vi "example_microFPGA_TTL.vi"() -> ()   [LabVIEW 2021]
panel:
  out "TTL_mode_READ":u16(ring)=1 items=["LO", "HIGH"]
  in  "TTL_channel":u16(ring)=3 items=["channel No 0", "channel No 1", "channel No 2", "channel No 3"]
  in  "write or read":u16(ring)=1 items=["read", "write"]
  out "value confirm":bool
  out "Version":u16=3
  in  "TTL_channel_WRITE":u16(ring)=1 items=["LO", "HIGH"]
  in  "close Application":bool=TRUE
  in  "send parameters":bool
  # "TTL control"
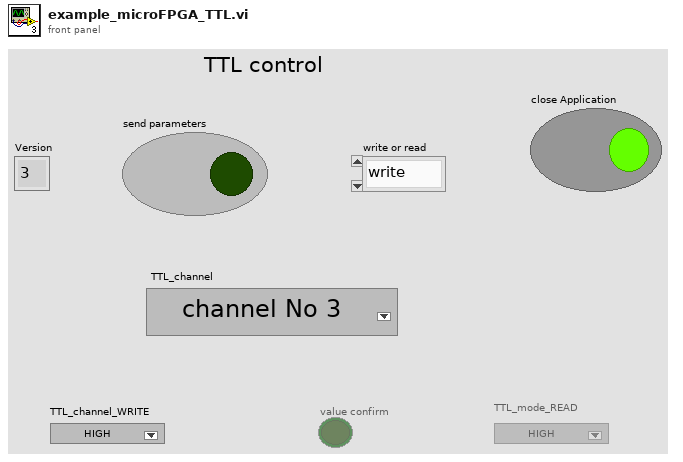
[diagram p1: front panel]
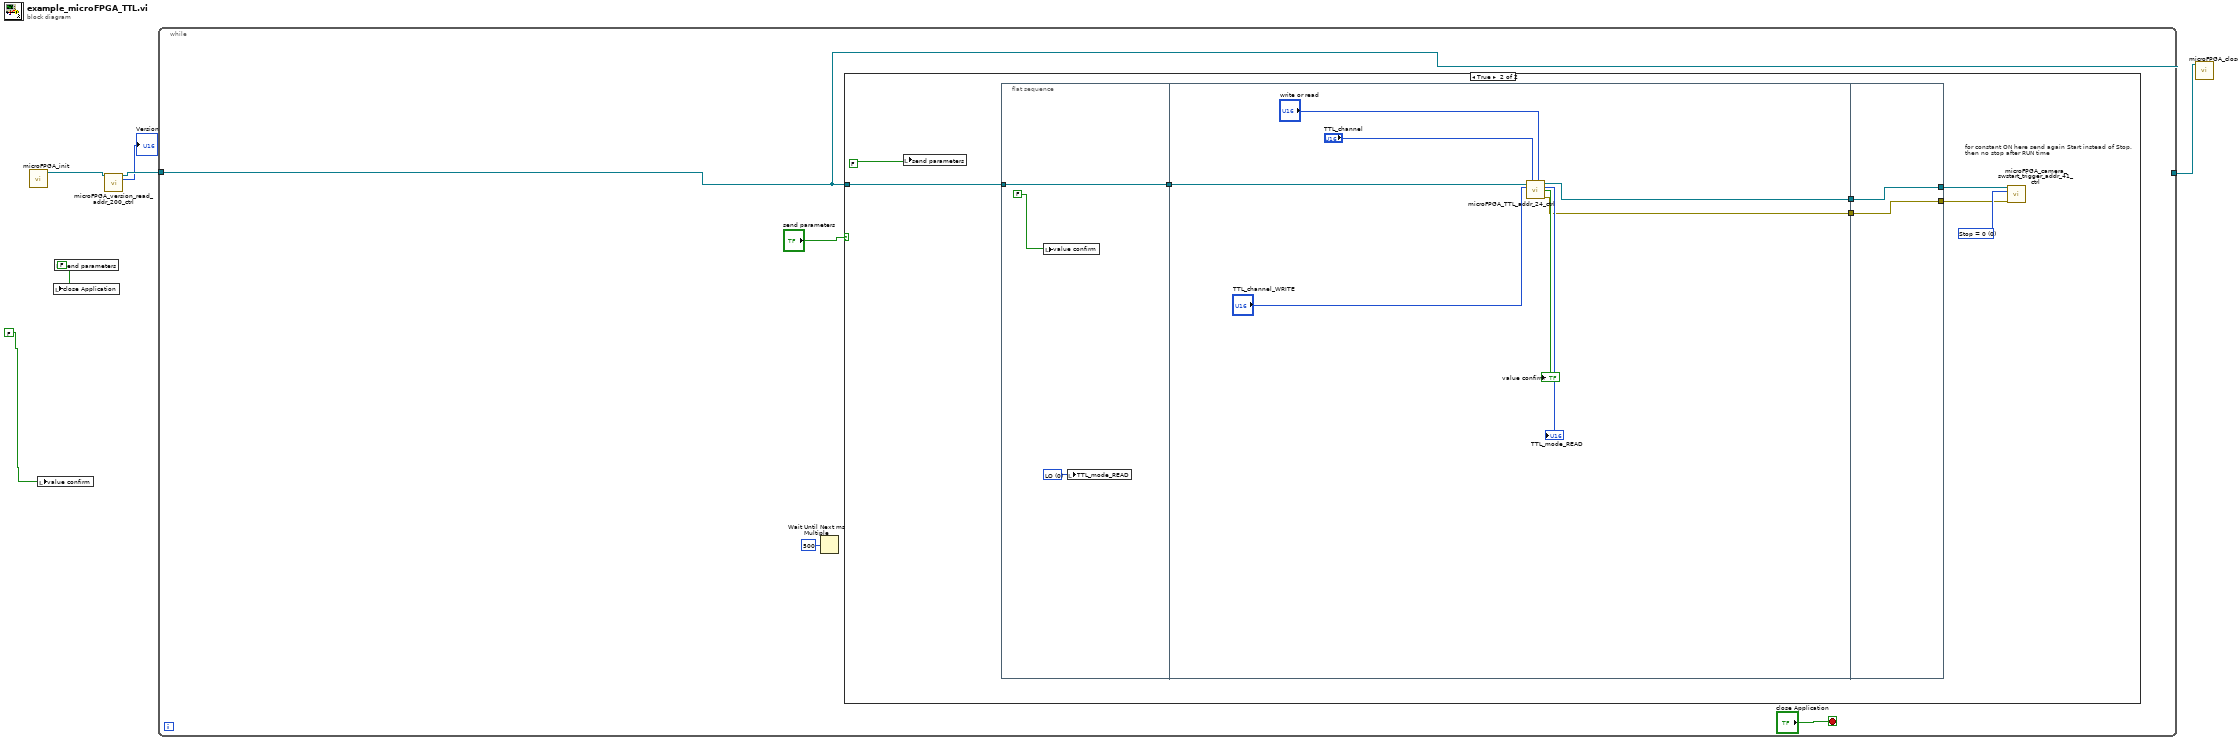
[diagram p0: block diagram]
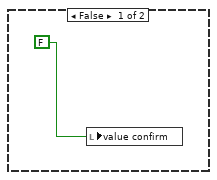
[diagram p2: hidden frame]
diagram:
  w6 = FALSE ("write")
  n1 = call "microFPGA_init.vi"() -> ("VISA resource name out"=w4:refnum<visa-resource-name>)  [unwired: 10 in, 1 out]
  n2 = local write "value confirm"(FALSE ("write")) -> ()
  n3 = local write "close Application"(w6) -> ()
  n4 = local write "send parameters"(w6) -> ()
  n5 = call "microFPGA_version_read_addr_200_ctrl.vi"("VISA resource name"=w4) -> ("VISA resource name 2"=w3:refnum<visa-resource-name>, "Version"=→"Version":u16)  [unwired: 12 in, 1 out]
  n6 = while {
    tunnel: w3 -> [w7]
    tunnel: [w7] -> w5
    stop <- "close Application" stop-if-true
    n7 = Wait Until Next ms Multiple(millisecond multiple=u32 500) -> ()  [unwired: 1 out]
    n8 = case shown="True" "send parameters" {
      tunnel: w7 -> [_ w18]
      frame False {
        n9 = local write "value confirm"(FALSE ("value write confirm")) -> ()
      }
      frame True {
        w16 = u16 0 items=["Stop = 0", "Start = 1 "] ("Camera_sw_start_WRITE 2")
        # "for constant ON here send again Start instead of Stop. \nthen no stop after RUN time"
        n10 = local write "send parameters"(FALSE ("write")) -> ()
        n11 = flat-sequence {
          tunnel: w18 -> [w22]
          tunnel: [w22] -> w17
          tunnel: w17 -> [w25]
          tunnel: [w24] -> w14
          tunnel: [w23] -> w13
          tunnel: [w32] -> w15
          tunnel: w14 -> [w32]
          tunnel: w13 -> [w31]
          tunnel: [w31] -> w12
          frame #0 {
            w21 = u16 0 items=["LO", "HIGH"] ("TTL_mode_READ")
            n12 = local write "value confirm"(FALSE ("value write confirm")) -> ()
            n13 = local write "TTL_mode_READ"(w21) -> ()
          }
          frame #1 {
            n14 = call "microFPGA_TTL_addr_24_ctrl.vi"("VISA resource name"=w25, "TTL_channel"="TTL_channel", "write or read"="write or read", "TTL_mode_WRITE"="TTL_channel_WRITE") -> ("VISA out"=w24:refnum<visa-resource-name>, "TTL_mode_READ"=→"TTL_mode_READ":u16, "value confirm"=→"value confirm":bool, "error out"=w23:errorcluster)  [unwired: 7 in, 1 out]
          }
          frame #2 {
          }
        }
        n15 = call "microFPGA_camera_swstart_trigger_addr_41_ctrl.vi"("VISA resource name"=w15, "Camera_sw_start_WRITE"=w16, "error in (no error)"=w12) -> ()  [unwired: 8 in, 5 out]
      }
    }
  }
  n16 = call "microFPGA_close.vi"("VISA resource name"=w5) -> ()  [unwired: 11 in]
